vi "Get_MeasControl.vi"(0 "FrontPanelData in":refnum<class "EpiWrapper.lvclass">, 1 "error in (no error)":errorcluster) -> (2 "FrontPanelData out":refnum<class "EpiWrapper.lvclass">, 3 "MeasureControl":refnum<vi>, 4 "error out":errorcluster)   [LabVIEW 2012, in "EpiWrapper.lvclass"]
uses:
  EpiWrapper.lvclass
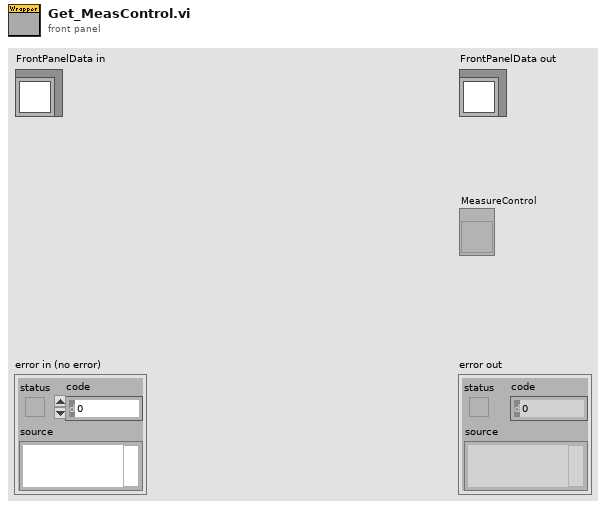
[diagram p1: front panel]
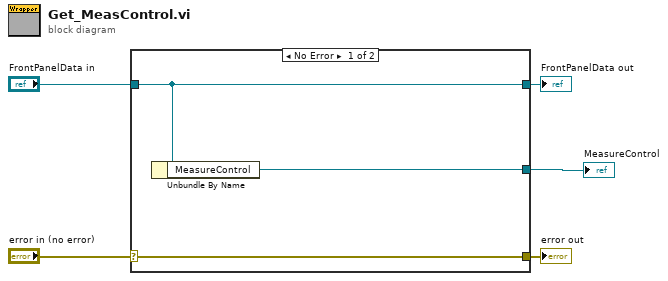
[diagram p0: block diagram]
diagram:
  n1 = case shown="No Error" "error in (no error)" {
    selector: "error in (no error)" -> [w8 w9]
    tunnel: [w8 w9] -> w4
    tunnel: [w7 w10] -> w2
    tunnel: "FrontPanelData in" -> [w7 w10]
    tunnel: [w6 _] -> w1
    frame No Error {
      n2 = Unbundle By Name(w7) -> ("MeasureControl"=w6:refnum<vi>)
    }
    frame Error {
    }
  }
  "error out" <- w4
  "FrontPanelData out" <- w2
  "MeasureControl" <- w1
